vi "GPIB Query.vi"(2 "Command String":string, 3 "Address":u16, 4 "VISA resource name":refnum<visa-resource-name>) -> (0 "Error":bool, 1 "Query Data":string)   [LabVIEW 2017]
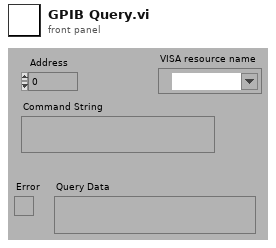
[diagram p1: front panel]
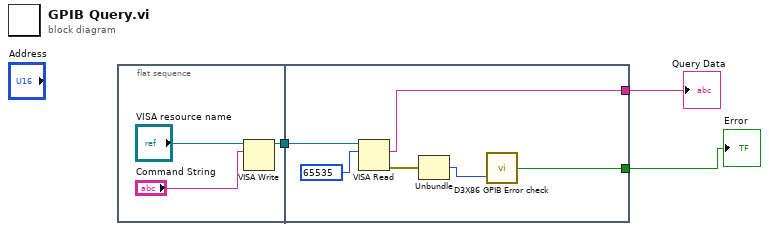
[diagram p0: block diagram]
diagram:
  n1 = flat-sequence {
    tunnel: [w4] -> w3
    tunnel: w3 -> [w12]
    tunnel: [w10] -> w2
    tunnel: [w7] -> w1
    frame #0 {
      n2 = VISA Write(VISA resource name="VISA resource name", write buffer="Command String") -> (VISA resource name out=w4:refnum<visa-resource-name>)  [unwired: 1 in, 2 out]
    }
    frame #1 {
      n3 = VISA Read(VISA resource name=w12, byte count=u32 65535) -> (read buffer=w10:string, error out=w9:errorcluster)  [unwired: 1 in, 2 out]
      n4 = Unbundle(w9) -> ("code"=w8:i32)  [unwired: 2 out]
      n5 = call "D3X86 GPIB Error check.vi"("GPIB Error"=w8) -> ("Error"=w7:bool)  [unwired: 1 in]
    }
  }
  "Error" <- w1
  "Query Data" <- w2
